vi "YKMW100 DO.vi"(0 "VISA session":refnum<visa-resource-name>="MW100", 5 "P1 - Channel":string="041", 7 "Relay Status (0:CLOSED)":enum8{"CLOSED", "OPEN"}(ring), 11 "error in (no error)":errorcluster) -> (4 "dup VISA session":refnum<visa-resource-name>="MW100", 15 "error out":errorcluster)   [LabVIEW 2016]
doc: "This VI changes the operation mode.\nThe effective operation mode is Setting Mode and Measurement Mode.\n\nSee also: command \"DS\"."
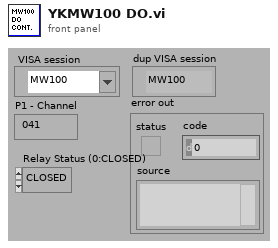
[diagram p1: front panel]
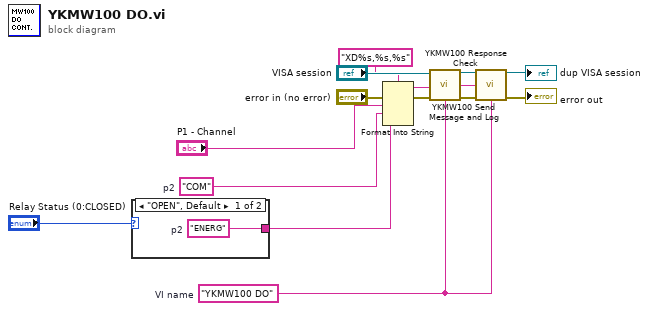
[diagram p0: block diagram]
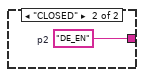
[diagram p2: hidden frame]
diagram:
  w3 = "COM"  # p2
  w5 = "YKMW100 DO"  # VI name
  n1 = case shown="\"OPEN\", Default" "Relay Status (0:CLOSED)" {
    tunnel: [w16 w17] -> w2
    frame "OPEN", Default {
      w16 = "ENERG"  # p2
    }
    frame "CLOSED" {
      w17 = "DE_EN"  # p2
    }
  }
  n2 = Format Into String(format string="XD%s,%s,%s", error in="error in (no error)", "P1 - Channel", w3, w2) -> (resulting string=w11:string, error out=w13:errorcluster)  [unwired: 1 in]
  n3 = call "YKMW100 Send Message and Log.vi"("VISA session"="VISA session", "Send Message (\"\")"=w11, "error in (no error)"=w13, "Source (\"\")"=w5) -> ("dup VISA session"=w10:refnum<visa-resource-name>, "Read Buffer"=w8:string, "error out"=w9:errorcluster)  [unwired: 9 in]
  n4 = call "YKMW100 Response Check.vi"("VISA session"=w10, "Message In (\"\")"=w8, "error in (no error)"=w9, "Source (\"\")"=w5) -> ("dup VISA session"=→"dup VISA session":refnum<visa-resource-name>, "error out"=→"error out":errorcluster)  [unwired: 7 in, 3 out]
